vi "update_faux_worm_set.vi"(5 "Worms to Draw":T1[](array[typedef])) -> (2 "Worms to Draw Updated":T1[](array[typedef]))   [LabVIEW 2019]
uses:
  FauxWorm.ctl
  <vilib>/numeric/Random Number (Range) I64.vi
  <vilib>/numeric/sub_Random U32.vi
  ParametersGlobal.vi
  <vilib>/ptbypt/NI_PtbyPt.lvlib
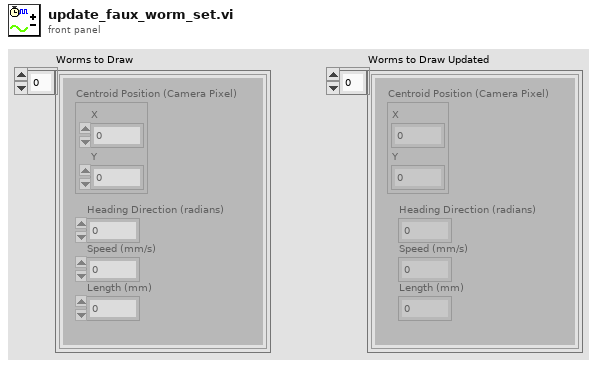
[diagram p1: front panel]
types:
  T1 = typedef "FauxWorm.ctl" = cluster{"Centroid Position (Camera Pixel)":cluster{"X":sgl, "Y":sgl}, "Heading Direction (radians)":dbl, "Speed (mm/s)":sgl, "Length (mm)":sgl}
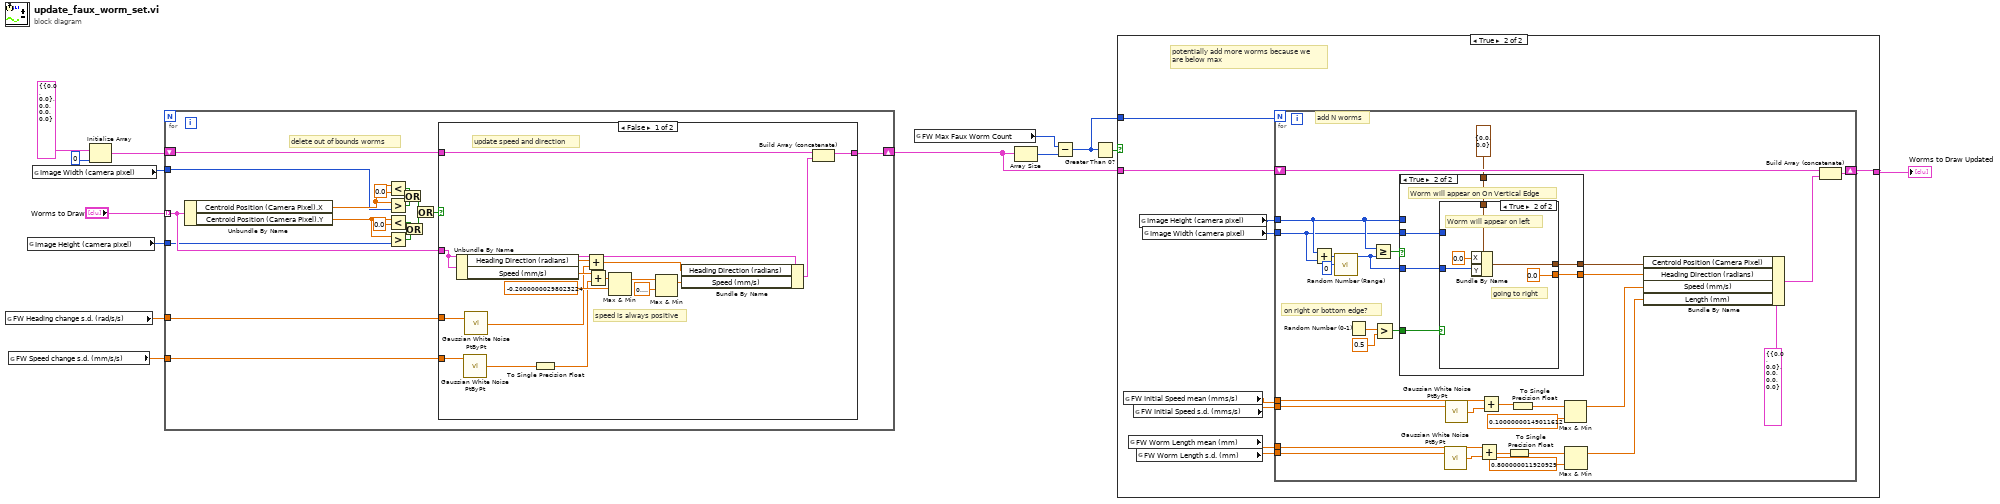
[diagram p0: block diagram]
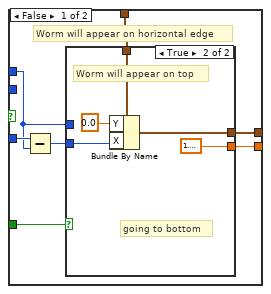
[diagram p4: hidden frame]
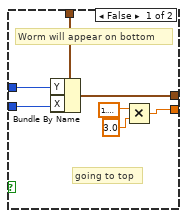
[diagram p5: hidden frame]
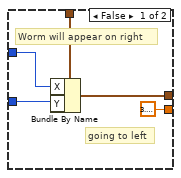
[diagram p6: hidden frame]
diagram:
  n1 = global read "ParametersGlobal.vi" "FW Heading change s.d. (rad/s/s)"() -> (w3:dbl)
  n2 = global read "ParametersGlobal.vi" "FW Speed change s.d. (mm/s/s)"() -> (w2:dbl)
  n3 = global read "ParametersGlobal.vi" "Image Height (camera pixel)"() -> (w4:i32)
  n4 = global read "ParametersGlobal.vi" "Image Width (camera pixel)"() -> (w5:i32)
  n5 = Initialize Array(T1 {"Centroid Position (Camera Pixel)"={"X"=0.0, "Y"=0.0}, "Heading Direction (radians)"=0.0, "Speed (mm/s)"=0.0, "Length (mm)"=0.0} ("Faux Worm Properties"), 0) -> (w10:T1[])
  n6 = for {
    tunnel: "Worms to Draw" -> [w21] mode=indexing
    shift-right: [w32] -> w9
    shift-left: w10 -> [w31]
    tunnel: w5 -> [w18]
    tunnel: w4 -> [w17]
    tunnel: w3 -> [w16]
    tunnel: w2 -> [w15]
    # "delete out of bounds worms"
    n7 = Unbundle By Name(w21) -> ("Centroid Position (Camera Pixel).X"=w20:sgl, "Centroid Position (Camera Pixel).Y"=w19:sgl)
    n8 = Less?(x=w20, y=sgl 0.0) -> (x < y?=w28:bool)
    n9 = Greater?(x=w20, y=w18) -> (0:w27:bool)
    n10 = Less?(x=w19, y=sgl 0.0) -> (x < y?=w26:bool)
    n11 = Greater?(x=w19, y=w17) -> (0:w25:bool)
    n12 = Or(x=w28, y=w27) -> (x .or. y?=w24:bool)
    n13 = Or(x=w26, y=w25) -> (x .or. y?=w23:bool)
    n14 = Or(x=w24, y=w23) -> (x .or. y?=w22:bool)
    n15 = case shown="False" w22 {
      tunnel: [w49 w50] -> w32
      tunnel: w31 -> [w48 w50]
      tunnel: w21 -> [w46 _]
      tunnel: w16 -> [w37 _]
      tunnel: w15 -> [w39 _]
      frame False {
        # "speed is always positive"
        # "update speed and direction"
        n16 = Unbundle By Name(w46) -> ("Heading Direction (radians)"=w45:dbl, "Speed (mm/s)"=w43:sgl)
        n17 = call <vilib>:"Gaussian White Noise PtByPt.vi"("standard deviation"=w39) -> ("Gaussian white noise"=w38:dbl)  [unwired: 2 in]
        n18 = call <vilib>:"Gaussian White Noise PtByPt.vi"("standard deviation"=w37) -> ("Gaussian white noise"=w36:dbl)  [unwired: 2 in]
        n19 = To Single Precision Float(number=w38) -> (single precision float=w40:sgl)
        n20 = Add(x=w45, y=w36) -> (x+y=w44:dbl)
        n21 = Add(x=w43, y=w40) -> (x+y=w41:sgl)
        n22 = Max & Min(x=w41, y=sgl -0.2) -> (max(x,y)=w35:sgl)  [unwired: 1 out]
        n23 = Max & Min(x=w35, y=sgl 0.2 ("x")) -> (min(x,y)=w33:sgl)  [unwired: 1 out]
        n24 = Bundle By Name(cluster=w46, "Heading Direction (radians)"=w44, "Speed (mm/s)"=w33) -> (w47:T1)
        n25 = Build Array (concatenate)(w48, w47) -> (w49:T1[])
      }
      frame True {
        # "the faux worm is out of the FOV, delete"
      }
    }
  }
  n26 = global read "ParametersGlobal.vi" "FW Max Faux Worm Count"() -> (w1:i32)
  n27 = Array Size(array=w9) -> (size(s)=w14:i32)
  n28 = Subtract(x=w1, y=w14) -> (x-y=w6:i32)
  n29 = Greater Than 0?(x=w6) -> (x > 0?=w7:bool)
  n30 = case shown="True" w7 {
    tunnel: w9 -> [w51 w60]
    tunnel: [w51 w59] -> w8
    tunnel: w6 -> [_ w52]
    frame False {
    }
    frame True {
      # "potentially add more worms because we\nare below max"
      n31 = global read "ParametersGlobal.vi" "FW Initial Speed mean (mms/s)"() -> (w53:dbl)
      n32 = global read "ParametersGlobal.vi" "FW Worm Length mean (mm)"() -> (w55:dbl)
      n33 = global read "ParametersGlobal.vi" "FW Initial Speed s.d. (mms/s)"() -> (w54:dbl)
      n34 = global read "ParametersGlobal.vi" "FW Worm Length s.d. (mm)"() -> (w56:dbl)
      n35 = global read "ParametersGlobal.vi" "Image Height (camera pixel)"() -> (w58:i32)
      n36 = global read "ParametersGlobal.vi" "Image Width (camera pixel)"() -> (w57:i32)
      n37 = for {
        N: w52 -> [_]
        shift-right: [w89] -> w59
        shift-left: w60 -> [w90]
        tunnel: w58 -> [w73]
        tunnel: w57 -> [w72]
        tunnel: w56 -> [w65]
        tunnel: w55 -> [w62]
        tunnel: w54 -> [w69]
        tunnel: w53 -> [w67]
        # "on right or bottom edge?"
        # "add N worms"
        n38 = Add(x=w73, y=w72) -> (x+y=w87:i32)
        n39 = call-poly <vilib>:"Random Number (Range).vi"("lower bound (-100)"=0, "upper bound (100)"=w87) -> ("number"=w83:i64)  [unwired: 9 in]
        n40 = Random Number (0-1)() -> (number: 0 to 1=w86:dbl)
        n41 = Greater Or Equal?(x=w73, y=w83) -> (x >= y?=w84:bool)
        n42 = Greater?(x=w86, y=0.5) -> (0:w82:bool)
        n43 = case shown="True" w84 {
          tunnel: w83 -> [w95 w114]
          tunnel: w73 -> [w91 _]
          tunnel: w72 -> [_ w111]
          tunnel: w82 -> [w96 w115]
          tunnel: cluster{"X":sgl, "Y":sgl} {"X"=0.0, "Y"=0.0} ("Centroid Position (Camera Pixel)") -> [w97 w113]
          tunnel: [w94 w112] -> w80
          tunnel: [w93 w110] -> w79
          frame False {
            # "Worm will appear on horizontal edge"
            n44 = Subtract(x=w95, y=w91) -> (x-y=w92:i64)
            n45 = case shown="True" w96 {
              tunnel: w97 -> [w104 w109]
              tunnel: [w103 w108] -> w94
              tunnel: [w98 1.5707963267948966] -> w93
              tunnel: w92 -> [w102 w106]
              tunnel: w91 -> [w101 _]
              frame False {
                # "going to top"
                # "Worm will appear on bottom"
                n46 = Bundle By Name(cluster=w104, "Y"=w101, "X"=w102) -> (w103:cluster{"X":sgl, "Y":sgl})
                n47 = Multiply(x=1.5707963267948966, y=3.0) -> (x*y=w98:dbl)
              }
              frame True {
                # "going to bottom"
                # "Worm will appear on top"
                n48 = Bundle By Name(cluster=w109, "Y"=sgl 0.0, "X"=w106) -> (w108:cluster{"X":sgl, "Y":sgl})
              }
            }
          }
          frame True {
            # "Worm will appear on On Vertical Edge"
            n49 = case shown="True" w115 {
              tunnel: w114 -> [w118 w124]
              tunnel: w113 -> [w120 w125]
              tunnel: [w119 w122] -> w112
              tunnel: w111 -> [w117 _]
              tunnel: [3.141592653589793 0.0] -> w110
              frame False {
                # "going to left"
                # "Worm will appear on right"
                n50 = Bundle By Name(cluster=w120, "X"=w117, "Y"=w118) -> (w119:cluster{"X":sgl, "Y":sgl})
              }
              frame True {
                # "going to right"
                # "Worm will appear on left"
                n51 = Bundle By Name(cluster=w125, "X"=sgl 0.0, "Y"=w124) -> (w122:cluster{"X":sgl, "Y":sgl})
              }
            }
          }
        }
        n52 = call <vilib>:"Gaussian White Noise PtByPt.vi"("standard deviation"=w65) -> ("Gaussian white noise"=w64:dbl)  [unwired: 2 in]
        n53 = call <vilib>:"Gaussian White Noise PtByPt.vi"("standard deviation"=w69) -> ("Gaussian white noise"=w68:dbl)  [unwired: 2 in]
        n54 = Add(x=w62, y=w64) -> (x+y=w63:dbl)
        n55 = Add(x=w67, y=w68) -> (x+y=w66:dbl)
        n56 = To Single Precision Float(number=w63) -> (single precision float=w70:sgl)
        n57 = To Single Precision Float(number=w66) -> (single precision float=w71:sgl)
        n58 = Max & Min(x=w71, y=sgl 0.1) -> (max(x,y)=w61:sgl)  [unwired: 1 out]
        n59 = Max & Min(x=w70, y=sgl 0.8) -> (max(x,y)=w76:sgl)  [unwired: 1 out]
        n60 = Bundle By Name(cluster=T1 {"Centroid Position (Camera Pixel)"={"X"=0.0, "Y"=0.0}, "Heading Direction (radians)"=0.0, "Speed (mm/s)"=0.0, "Length (mm)"=0.0} ("Faux Worm Properties"), "Centroid Position (Camera Pixel)"=w80, "Heading Direction (radians)"=w79, "Speed (mm/s)"=w61, "Length (mm)"=w76) -> (w75:T1)
        n61 = Build Array (concatenate)(w90, w75) -> (w89:T1[])
      }
    }
  }
  "Worms to Draw Updated" <- w8
